vi "set_config_cluster.vi"(8 "error in (no error)":errorcluster, 10 "config cluster variant":variant, 11 "LightSourceDL090903Laser in":refnum<class "LightSourceDL090903Laser.lvclass">) -> (0 "error out":errorcluster, 3 "LightSourceDL090903Laser out":refnum<class "LightSourceDL090903Laser.lvclass">)   [LabVIEW 2010, in "LightSourceDL090903Laser.lvclass"]
uses:
  LightSourceDL090903Laser.lvclass
  LightSourceDL090903Laser.lvclass/LightSourceDL090903Laser.ctl
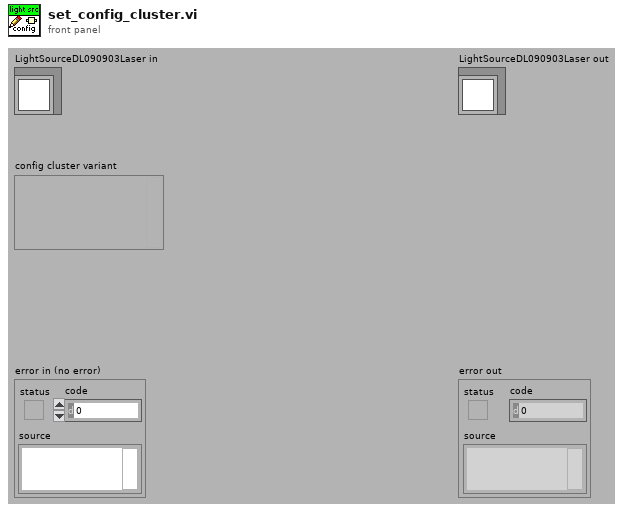
[diagram p1: front panel]
types:
  T1 = typedef "LightSourceDL090903Laser.lvclass/config_data_cluster.ctl" = cluster{"LSID":T2, "manufacturer specification":T3, "type":T4, "laser medium":T5, "frequency multiplication":dbl, "tuneable?":bool, "pulse":T6, "repetition rate":dbl[unit], "pump laser configuration":string}
  T2 = typedef "LSID_cluster.ctl" = cluster{"identifier":string, "revision":i32}
  T3 = typedef "GenericComponent.lvclass/manufacturer_specification_cluster.ctl" = cluster{"manufacturer":string, "model":string, "serial number":string, "lot number":string}
  T4 = typedef "LightSourceDL090903Laser.lvclass/type_enum.ctl" = enum16{"Excimer", "Gas", "MetalVapor", "SolidState", "Dye", "Semiconductor", "FreeElectron", "Unknown"}
  T5 = typedef "LightSourceDL090903Laser.lvclass/laser_medium_enum.ctl" = enum16{"Cu", "Ag", "ArFl", "ArCl", "KrFl", "XeFl", "XeCl", "XeBr", "N", "Ar", "Kr", "Xe", "HeNe", "HeCd", "CO", "CO2", "H2O", "HFl", "NdGlass", "NdYAG", "ErGlass", "ErYAG", "HoYLF", "HoYAG", "Ruby", "TiSapphire", "Alexandrite", "Rhodamine6G", "CoumarineC30", "GaAs", "GaAlAs", "EMinus", "Unknown"}
  T6 = typedef "LightSourceDL090903Laser.lvclass/pulse_enum.ctl" = enum16{"CW", "Single", "QSwitched", "Repetitive", "ModeLocked"}
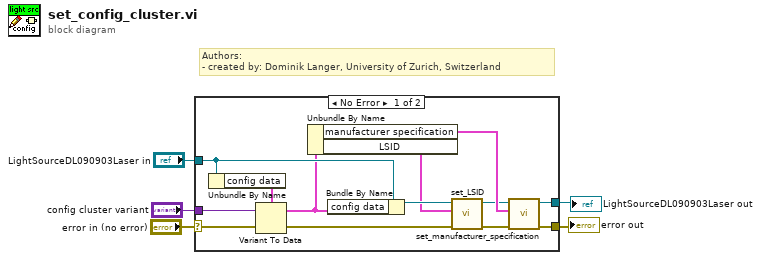
[diagram p0: block diagram]
diagram:
  # "Authors: \n- created by: Dominik Langer, University of Zurich, Switzerland"
  n1 = case shown="No Error" "error in (no error)" {
    selector: "error in (no error)" -> [w13 w20]
    tunnel: [w16 w20] -> w2
    tunnel: [w15 w19] -> w1
    tunnel: "LightSourceDL090903Laser in" -> [w12 w19]
    tunnel: "config cluster variant" -> [w14 _]
    frame No Error {
      n2 = Unbundle By Name(w12) -> ("config data"=w17:T1)
      n3 = Variant To Data(error in=w13, Variant=w14, type=w17) -> (error out=w18:errorcluster, data=w11:T1)
      n4 = Unbundle By Name(w11) -> ("manufacturer specification"=w8:T3, "LSID"=w9:T2)
      n5 = Bundle By Name(cluster=w12, "config data"=w11) -> (w10:refnum<class "LightSourceDL090903Laser.lvclass">)
      n6 = call-dynamic "set_LSID.vi"("error in (no error)"=w18, "LSID"=w9, "GenericPlugin in"=w10) -> ("error out"=w7:errorcluster, "GenericPlugin out"=w6:refnum<class "LightSourceDL090903Laser.lvclass">)  [unwired: 7 in]
      n7 = call-dynamic "set_manufacturer_specification.vi"("error in (no error)"=w7, "manufacturer specification"=w8, "GenericPlugin in"=w6) -> ("error out"=w16:errorcluster, "GenericPlugin out"=w15:refnum<class "LightSourceDL090903Laser.lvclass">)  [unwired: 7 in]
    }
    frame Error {
    }
  }
  "error out" <- w2
  "LightSourceDL090903Laser out" <- w1
